vi "addArgument_NumpyArray2d_Bool.vi"(7 "argument name":string, 8 "error in (no error)":errorcluster, 9 "argument list in":T1[](array[typedef]), 10 "Array":bool[][](array[boolean]), 11 "LabVIEW-Python-Interface in":refnum<class "PyLVi.lvclass">) -> (0 "error out":errorcluster, 1 "argument list out":T1[](array[typedef]), 3 "LabVIEW-Python-Interface out":refnum<class "PyLVi.lvclass">)   [LabVIEW 2016, in "PyLVi.lvlib" / "PyLVi.lvclass"]
uses:
  PyLVi.lvclass
  Controls/ArgumentStructure.ctl
  Controls/DescriptorStructure.ctl
  Controls/ArgumentType.ctl
  Controls/DataType.ctl
panel:
  out "data string":string
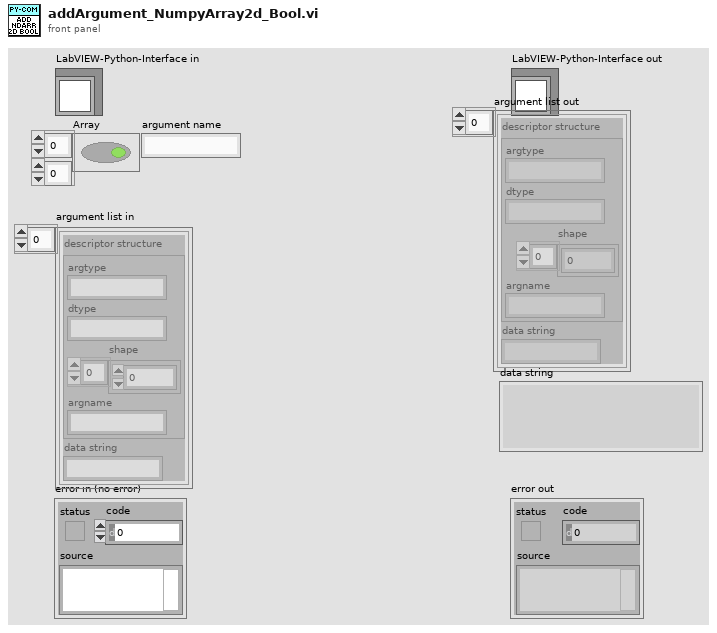
[diagram p1: front panel]
types:
  T1 = typedef "PyLVi.lvlib/PyLVi.lvclass/ArgumentStructure.ctl" = cluster{"descriptor structure":T2, "data string":string}
  T2 = typedef "PyLVi.lvlib/PyLVi.lvclass/DescriptorStructure.ctl" = cluster{"argtype":string, "dtype":string, "shape":u32[], "argname":string}
  T3 = enum16{"big-endian, network order", "native, host order", "little-endian"}
  T4 = typedef "PyLVi.lvlib/PyLVi.lvclass/DataType.ctl" = enum16{"bool", "string", "int16", "int32", "float32", "float64", "complex128"}
  T5 = typedef "PyLVi.lvlib/PyLVi.lvclass/ArgumentType.ctl" = enum8{"bool", "numeric", "string", "dict", "ndarray", "ndarray2d"}
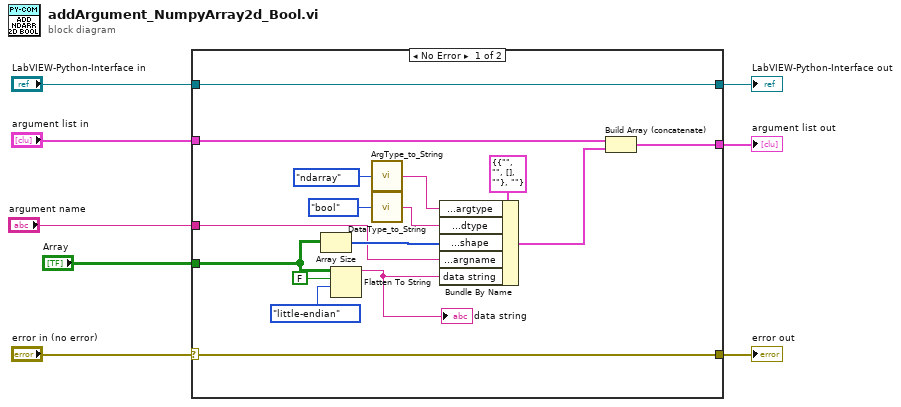
[diagram p0: block diagram]
diagram:
  n1 = case shown="No Error" "error in (no error)" {
    selector: "error in (no error)" -> [w24 w26]
    tunnel: [w24 w26] -> w7
    tunnel: [w23 w27] -> w5
    tunnel: "LabVIEW-Python-Interface in" -> [w23 w27]
    tunnel: "Array" -> [w16 _]
    tunnel: "argument list in" -> [w21 w25]
    tunnel: [w19 w25] -> w3
    tunnel: "argument name" -> [w9 _]
    frame No Error {
      n2 = Array Size(array=w16) -> (size(s)=w10:i32[])
      n3 = Flatten To String(anything=w16, prepend array or string size? (T)=FALSE, byte order (0:big-endian, network order)=T3."little-endian") -> (data string=w15:string)  [unwired: 1 in, 2 out]
      "data string" <- w15
      n4 = call "ArgType_to_String.vi"("arg type"=ArgumentType."ndarray" ("descriptor structure.argtype")) -> ("arg type string"=w12:string)  [unwired: 4 in]
      n5 = call "DataType_to_String.vi"("data type"=DataType."bool" ("descriptor structure.dtype")) -> ("data type string"=w11:string)  [unwired: 4 in]
      n6 = Bundle By Name(cluster=T1 {"descriptor structure"={"argtype"="", "dtype"="", "shape"=[], "argname"=""}, "data string"=""} ("argument structure"), "descriptor structure.argtype"=w12, "descriptor structure.dtype"=w11, "descriptor structure.shape"=w10, "descriptor structure.argname"=w9, "data string"=w15) -> (w20:T1)
      n7 = Build Array (concatenate)(w21, w20) -> (w19:T1[])
    }
    frame Error {
    }
  }
  "error out" <- w7
  "LabVIEW-Python-Interface out" <- w5
  "argument list out" <- w3
